vi "Quick Test V2.vi"() -> ()   [LabVIEW 2010]
uses:
  <vilib>/SwitchExecutive/nise.llb/niSE Multiconnect Mode Enum.ctl
panel:
  in  "Load All Channels":bool
  in  "DMM to DVDD":bool
  in  "SMU1 to VRECT":bool
  in  "stop":bool
  in  "SMU3 to VBAT + BATT SIM":bool
  in  "SMU3 to VBAT":bool
  in  "JTAG DVDD POWER":bool
  in  "JTAG DATA":bool
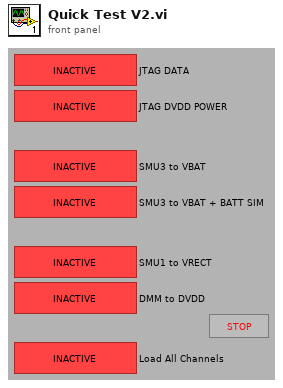
[diagram p1: front panel]
types:
  T1 = typedef "niSE SessionRefnum.ctl" = refnum<k1>
  T2 = enum16{"--Disconnect All--", "Connect PulseGen to CH1", "Connect PulseGen to CH2", "Connect PulseGen to CH3", "Connect PulseGen to CH4", "Connect PulseGen to CH5", "Connect PulseGen to CH6", "Connect PulseGen to CH7", "Connect PulseGen to CH8", "Connect PulseGen to CH9", "Connect PulseGen to CH10", "Connect PulseGen to CH11", "Connect PulseGen to CH12", "Connect PulseGen to CH13", "Connect PulseGen to CH14", "Connect PulseGen to CH15", "Connect PulseGen to CH16", "Connect PulseGen to CH17", "Connect PulseGen to CH18", "Connect PulseGen to CH19", "Connect PulseGen to CH20", "Connect PulseGen to CH21", "Connect PulseGen to CH22", "Connect PulseGen to CH23", "Connect PulseGen to CH24", "Connect PulseGen to CH25", "Set MAG_SW", "Set Dynamic Load", "Set Expansion Trigger", "Trigger Positive Pulse", "Trigger Negative Pulse", "Set MSP Magic Pin", "Set BAT_EN", "Connect MSP_ACLK to CTR", "Connect MSP_MCLK to CTR", "Connect MSP_DIG_TST_OUT to CTR", "Connect STIM_SCK to CTR", "Connect STIM_CLK to CTR", "Connect SMU2 to Magnet", "Magnet Enable", "Cap Short", "Connect Positive Pulse to Pulse Bus", "Connect Negative Pulse to Pulse Bus", "Connect JTAG", "Connect JTAG DVDD Power", "RF Attach", "Connect SMU3 to VBAT", "Connect SMU3 Soft Start", "Connect ARB to Charge Coil", "Connect ARB to Matrix", "Connect CTR to Matrix", "DMM_I Short", "DMM_I 1000 Ohm", "DMM_I 100 Ohm", "DMM_I 10 Ohm", "Connect CH25 to DUT GND"}
  T3 = typedef "niSE Multiconnect Mode Enum.ctl" = i32
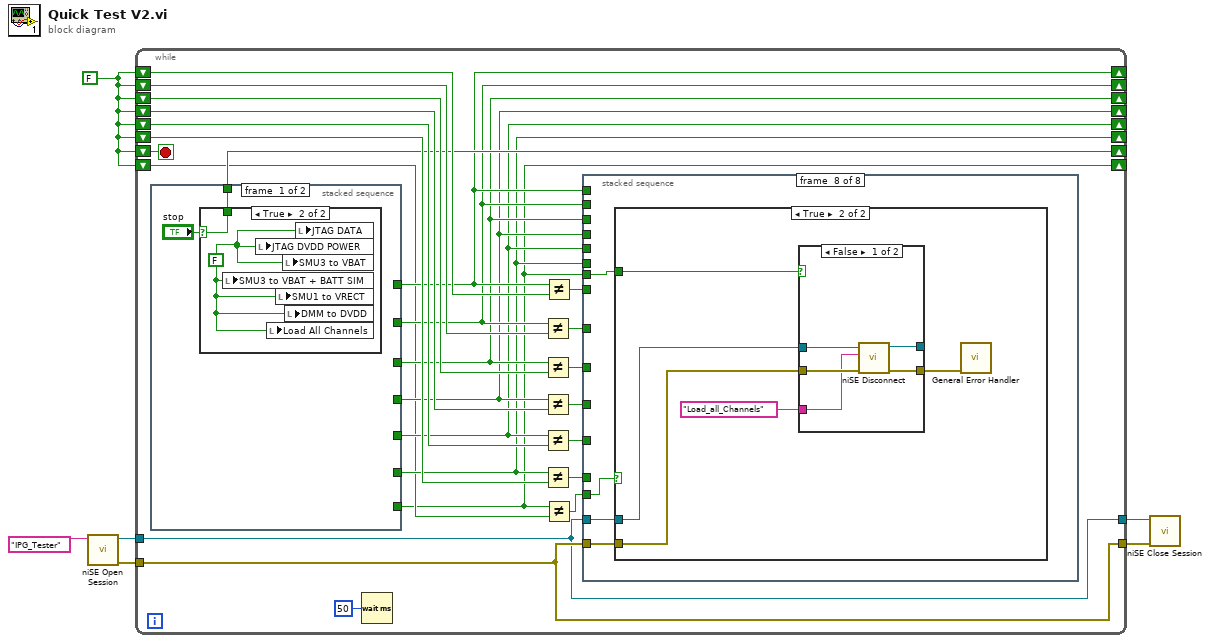
[diagram p0: block diagram]
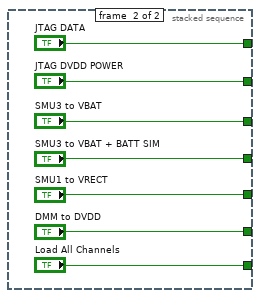
[diagram p3: hidden frame]
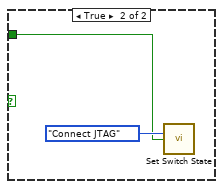
[diagram p6: hidden frame]
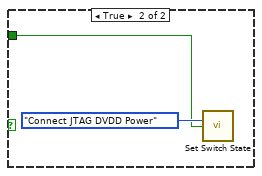
[diagram p8: hidden frame]
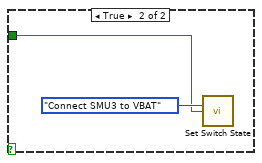
[diagram p10: hidden frame]
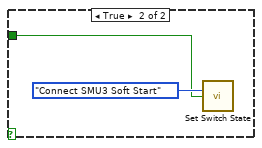
[diagram p12: hidden frame]
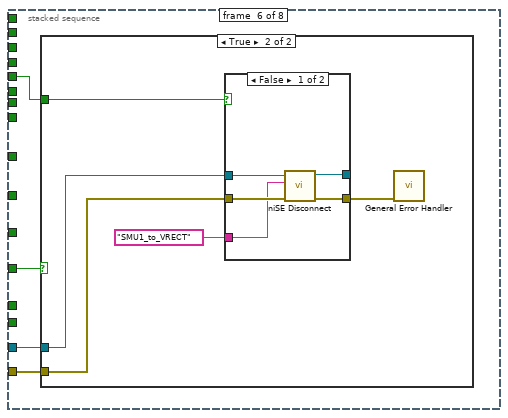
[diagram p13: hidden frame]
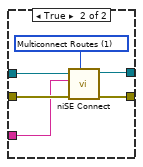
[diagram p15: hidden frame]
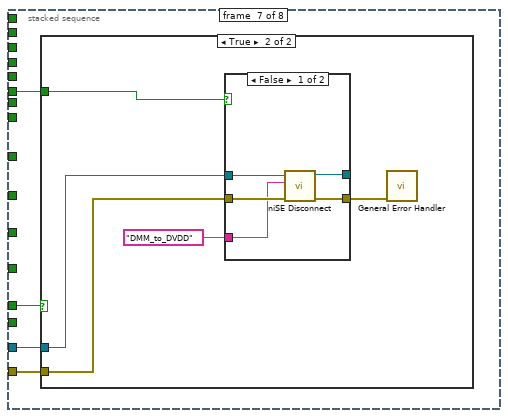
[diagram p16: hidden frame]
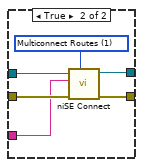
[diagram p18: hidden frame]
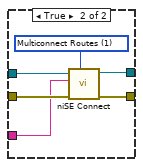
[diagram p20: hidden frame]
diagram:
  w1 = FALSE
  n1 = call <vilib>:"niSE Open Session.vi"("Virtual Device Name (SwitchConfiguration1)"="IPG_Tester") -> ("error out"=w4:errorcluster, "NISE Session (out)"=w5:T1)  [unwired: 5 in]
  n2 = while {
    shift-right: [w15] -> _
    shift-left: w1 -> [w32]
    shift-right: [w14] -> _
    shift-left: w1 -> [w31]
    shift-right: [w13] -> _
    shift-left: w1 -> [w30]
    shift-right: [w12] -> _
    shift-left: w1 -> [w29]
    shift-right: [w11] -> _
    shift-left: w1 -> [w21]
    shift-right: [w10] -> _
    shift-left: w1 -> [w20]
    tunnel: w5 -> [w18]
    tunnel: w4 -> [w19]
    tunnel: [w18] -> w3
    tunnel: [w19] -> w2
    shift-right: [w16] -> _
    shift-left: w1 -> [w17]
    shift-right: [w7] -> _
    shift-left: w1 -> [w9]
    stop <- w17 stop-if-true
    n3 = stacked-sequence {
      tunnel: [w33 _] -> w16
      tunnel: [_ "JTAG DATA"] -> w15
      tunnel: [_ "JTAG DVDD POWER"] -> w14
      tunnel: [_ "SMU3 to VBAT"] -> w13
      tunnel: [_ "SMU3 to VBAT + BATT SIM"] -> w12
      tunnel: [_ "SMU1 to VRECT"] -> w11
      tunnel: [_ "DMM to DVDD"] -> w10
      tunnel: [_ "Load All Channels"] -> w7
      frame #0 {
        n4 = case shown="True" "stop" {
          selector: "stop" -> [w35 w37]
          tunnel: [w35 w37] -> w33
          frame False {
          }
          frame True {
            w36 = FALSE
            n5 = local write "SMU3 to VBAT + BATT SIM"(w36) -> ()
            n6 = local write "JTAG DVDD POWER"(w36) -> ()
            n7 = local write "Load All Channels"(w36) -> ()
            n8 = local write "SMU1 to VRECT"(w36) -> ()
            n9 = local write "SMU3 to VBAT"(w36) -> ()
            n10 = local write "DMM to DVDD"(w36) -> ()
            n11 = local write "JTAG DATA"(w36) -> ()
          }
        }
      }
      frame #1 {
      }
    }
    n12 = Wait (ms)(milliseconds to wait=u32 50) -> ()  [unwired: 1 out]
    n13 = Not Equal?(x=w14, y=w31) -> (x != y?=w27:bool)
    n14 = Not Equal?(x=w13, y=w30) -> (x != y?=w26:bool)
    n15 = Not Equal?(x=w12, y=w29) -> (x != y?=w25:bool)
    n16 = Not Equal?(x=w11, y=w21) -> (x != y?=w23:bool)
    n17 = Not Equal?(x=w10, y=w20) -> (x != y?=w22:bool)
    n18 = Not Equal?(x=w15, y=w32) -> (x != y?=w28:bool)
    n19 = Not Equal?(x=w7, y=w9) -> (x != y?=w8:bool)
    n20 = stacked-sequence {
      tunnel: w12 -> [_ _ _ _ w57 _ _ _]
      tunnel: w13 -> [_ _ _ w53 _ _ _ _]
      tunnel: w14 -> [_ _ w50 _ _ _ _ _]
      tunnel: w15 -> [_ w46 _ _ _ _ _ _]
      tunnel: w28 -> [_ w45 _ _ _ _ _ _]
      tunnel: w27 -> [_ _ w49 _ _ _ _ _]
      tunnel: w26 -> [_ _ _ w54 _ _ _ _]
      tunnel: w25 -> [_ _ _ _ w58 _ _ _]
      tunnel: w23 -> [_ _ _ _ _ w64 _ _]
      tunnel: w22 -> [_ _ _ _ _ _ w83 _]
      tunnel: w11 -> [_ _ _ _ _ w63 _ _]
      tunnel: w10 -> [_ _ _ _ _ _ w84 _]
      tunnel: w18 -> [_ _ _ _ _ w61 w82 w104]
      tunnel: w19 -> [_ _ _ _ _ w62 w81 w103]
      tunnel: w8 -> [_ _ _ _ _ _ _ w102]
      tunnel: w7 -> [_ _ _ _ _ _ _ w101]
      frame #0 {
      }
      frame #1 {
        n21 = case shown="False" w45 {
          tunnel: w46 -> [_ w47]
          frame False {
          }
          frame True {
            n22 = call "Set Switch State.vi"("Action"=T2."Connect JTAG", "State"=w47) -> ()  [unwired: 13 in, 1 out]
          }
        }
      }
      frame #2 {
        n23 = case shown="False" w49 {
          tunnel: w50 -> [_ w51]
          frame False {
          }
          frame True {
            n24 = call "Set Switch State.vi"("Action"=T2."Connect JTAG DVDD Power", "State"=w51) -> ()  [unwired: 13 in, 1 out]
          }
        }
      }
      frame #3 {
        n25 = case shown="False" w54 {
          tunnel: w53 -> [_ w55]
          frame False {
          }
          frame True {
            n26 = call "Set Switch State.vi"("Action"=T2."Connect SMU3 to VBAT", "State"=w55) -> ()  [unwired: 13 in, 1 out]
          }
        }
      }
      frame #4 {
        n27 = case shown="False" w58 {
          tunnel: w57 -> [_ w59]
          frame False {
          }
          frame True {
            n28 = call "Set Switch State.vi"("Action"=T2."Connect SMU3 Soft Start", "State"=w59) -> ()  [unwired: 13 in, 1 out]
          }
        }
      }
      frame #5 {
        n29 = case shown="True" w64 {
          tunnel: w63 -> [_ w69]
          tunnel: w62 -> [_ w67]
          tunnel: w61 -> [_ w66]
          frame False {
          }
          frame True {
            n30 = case shown="False" w69 {
              tunnel: w66 -> [w74 w78]
              tunnel: [w73 w80] -> w65
              tunnel: w67 -> [w72 w79]
              tunnel: [w71 w77] -> _
              tunnel: "SMU1_to_VRECT" ("Virtual Device Name (SwitchConfiguration1)") -> [w70 w76]
              frame False {
                n31 = call <vilib>:"niSE Disconnect.vi"("error in (no error)"=w72, "Disconnection Specification (\"\")"=w70, "NISE Session (in)"=w74) -> ("error out"=w73:errorcluster, "NISE Session (out)"=w71:T1)  [unwired: 3 in]
              }
              frame True {
                w75 = T3 1 items=["Use Default Mode"=-1, "Multiconnect Routes"=1, "No Multiconnect"=0] ("Multiconnect Mode (Use Default Mode)")
                n32 = call <vilib>:"niSE Connect.vi"("Multiconnect Mode (Use Default Mode)"=w75, "error in (no error)"=w79, "Connection Specification (\"\")"=w76, "NISE Session (in)"=w78) -> ("error out"=w80:errorcluster, "NISE Session (out)"=w77:T1)  [unwired: 6 in]
              }
            }
            n33 = call <vilib>:"General Error Handler.vi"("error in (no error)"=w65) -> ()  [unwired: 10 in, 5 out]
          }
        }
      }
      frame #6 {
        n34 = case shown="True" w83 {
          tunnel: w84 -> [_ w89]
          tunnel: w82 -> [_ w87]
          tunnel: w81 -> [_ w86]
          frame False {
          }
          frame True {
            n35 = case shown="False" w89 {
              tunnel: w87 -> [w94 w98]
              tunnel: [w93 w100] -> w85
              tunnel: w86 -> [w92 w99]
              tunnel: [w91 w97] -> _
              tunnel: "DMM_to_DVDD" ("Virtual Device Name (SwitchConfiguration1)") -> [w90 w96]
              frame False {
                n36 = call <vilib>:"niSE Disconnect.vi"("error in (no error)"=w92, "Disconnection Specification (\"\")"=w90, "NISE Session (in)"=w94) -> ("error out"=w93:errorcluster, "NISE Session (out)"=w91:T1)  [unwired: 3 in]
              }
              frame True {
                w95 = T3 1 items=["Use Default Mode"=-1, "Multiconnect Routes"=1, "No Multiconnect"=0] ("Multiconnect Mode (Use Default Mode)")
                n37 = call <vilib>:"niSE Connect.vi"("Multiconnect Mode (Use Default Mode)"=w95, "error in (no error)"=w99, "Connection Specification (\"\")"=w96, "NISE Session (in)"=w98) -> ("error out"=w100:errorcluster, "NISE Session (out)"=w97:T1)  [unwired: 6 in]
              }
            }
            n38 = call <vilib>:"General Error Handler.vi"("error in (no error)"=w85) -> ()  [unwired: 10 in, 5 out]
          }
        }
      }
      frame #7 {
        n39 = case shown="True" w102 {
          tunnel: w101 -> [_ w109]
          tunnel: w104 -> [_ w107]
          tunnel: w103 -> [_ w106]
          frame False {
          }
          frame True {
            n40 = case shown="False" w109 {
              tunnel: w107 -> [w114 w118]
              tunnel: [w113 w120] -> w105
              tunnel: w106 -> [w112 w119]
              tunnel: [w111 w117] -> _
              tunnel: "Load_all_Channels" ("Virtual Device Name (SwitchConfiguration1)") -> [w110 w116]
              frame False {
                n41 = call <vilib>:"niSE Disconnect.vi"("error in (no error)"=w112, "Disconnection Specification (\"\")"=w110, "NISE Session (in)"=w114) -> ("error out"=w113:errorcluster, "NISE Session (out)"=w111:T1)  [unwired: 3 in]
              }
              frame True {
                w115 = T3 1 items=["Use Default Mode"=-1, "Multiconnect Routes"=1, "No Multiconnect"=0] ("Multiconnect Mode (Use Default Mode)")
                n42 = call <vilib>:"niSE Connect.vi"("Multiconnect Mode (Use Default Mode)"=w115, "error in (no error)"=w119, "Connection Specification (\"\")"=w116, "NISE Session (in)"=w118) -> ("error out"=w120:errorcluster, "NISE Session (out)"=w117:T1)  [unwired: 6 in]
              }
            }
            n43 = call <vilib>:"General Error Handler.vi"("error in (no error)"=w105) -> ()  [unwired: 10 in, 5 out]
          }
        }
      }
    }
  }
  n44 = call <vilib>:"niSE Close Session.vi"("error in (no error)"=w2, "NISE Session (in)"=w3) -> ()  [unwired: 5 in, 1 out]
